vi "Bay_Enter_Exit_Timer.vi"(8 "reset button":bool) -> (0 "Indicator":dbl)   [LabVIEW 2024]
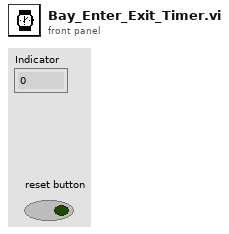
[diagram p1: front panel]
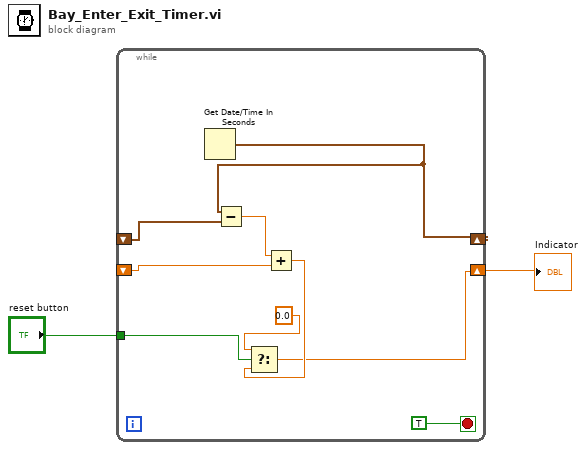
[diagram p0: block diagram]
diagram:
  n1 = while {
    shift-right: [w3] -> _
    shift-left: _ -> [w11]
    shift-right: [w4] -> w2
    shift-left: _ -> [w5]
    tunnel: "reset button" -> [w8]
    stop <- TRUE stop-if-true
    n2 = Get Date/Time In Seconds() -> (seconds since 1Jan1904=w3:timestamp)
    n3 = Subtract(x=w3, y=w11) -> (x-y=w10:dbl)
    n4 = Add(x=w10, y=w5) -> (x+y=w6:dbl)
    n5 = Select(t=0.0, s=w8, f=w6) -> (s? t:f=w4:dbl)
  }
  "Indicator" <- w2
